vi "Oszilloscope_init.vi"(8 "error in":errorcluster, 11 "VISA-Ressourcenname":refnum<visa-resource-name>="USB0::0x0957::0x179B::MY54313507::INSTR") -> (0 "error out 2":errorcluster)   [LabVIEW 2016]
doc: "Mit diesem VI wird das Oszilloscope DSO-X-2002A initialisiert."
uses:
  <instrlib>/Agilent 2000 3000 X-Series/Agilent 2000 3000 X-Series.lvlib
panel:
  in  "Vertikale Skalierung (0,015 V/div)":dbl=0.015
  in  "Zeit Skalierung (0.004 Sec/div)":dbl=0.004
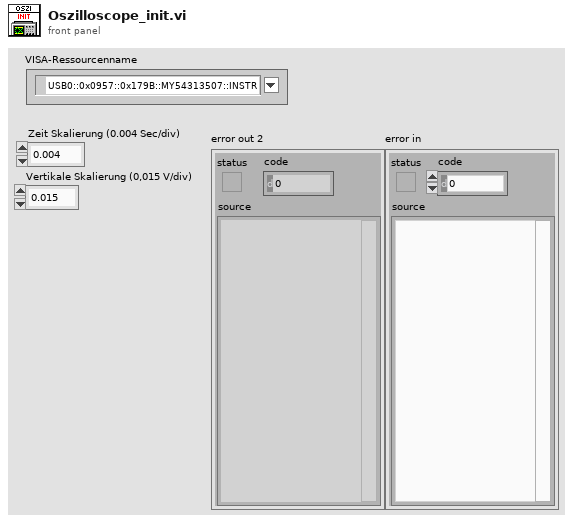
[diagram p1: front panel]
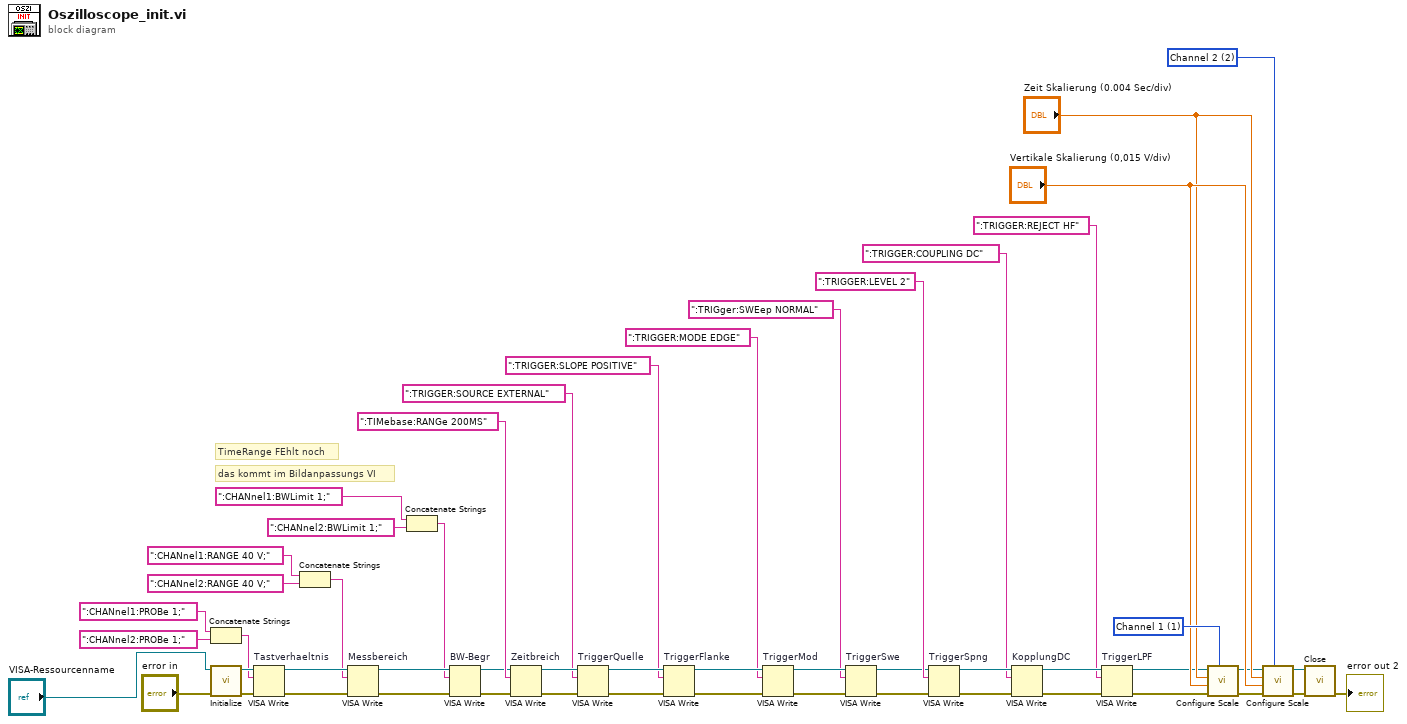
[diagram p0: block diagram]
diagram:
  w29 = 2 items=["Channel 1"=1, "Channel 2"=2, "Channel 3"=3, "Channel 4"=4] ("Channel Name (1: Channel 1)")
  w52 = 1 items=["Channel 1"=1, "Channel 2"=2, "Channel 3"=3, "Channel 4"=4] ("Channel Name (1: Channel 1)")
  # "das kommt im Bildanpassungs VI"
  # "TimeRange FEhlt noch"
  n1 = Concatenate Strings(":CHANnel1:PROBe 1;" ("Schreibpuffer"), ":CHANnel2:PROBe 1;" ("Schreibpuffer")) -> (w34:string)
  n2 = call <instrlib>:"Initialize.vi"("error in (no error)"="error in", "VISA resource name"="VISA-Ressourcenname") -> ("error out"=w48:errorcluster, "VISA resource name out"=w49:refnum<visa-resource-name>)  [unwired: 8 in]
  n3 = VISA Write "Tastverhaeltnis"(VISA resource name=w49, write buffer=w34, error in (no error)=w48) -> (VISA resource name out=w46:refnum<visa-resource-name>, error out=w43:errorcluster)  [unwired: 1 out]
  n4 = Concatenate Strings(":CHANnel1:RANGE 40 V;" ("Schreibpuffer"), ":CHANnel2:RANGE 40 V;" ("Schreibpuffer")) -> (w39:string)
  n5 = VISA Write "Messbereich"(VISA resource name=w46, write buffer=w39, error in (no error)=w43) -> (VISA resource name out=w45:refnum<visa-resource-name>, error out=w44:errorcluster)  [unwired: 1 out]
  n6 = Concatenate Strings(":CHANnel1:BWLimit 1;" ("Schreibpuffer"), ":CHANnel2:BWLimit 1;" ("Schreibpuffer")) -> (w40:string)
  n7 = VISA Write "BW-Begr"(VISA resource name=w45, write buffer=w40, error in (no error)=w44) -> (VISA resource name out=w28:refnum<visa-resource-name>, error out=w27:errorcluster)  [unwired: 1 out]
  n8 = VISA Write "Zeitbreich"(VISA resource name=w28, write buffer=":TIMebase:RANGe 200MS" ("Schreibpuffer"), error in (no error)=w27) -> (VISA resource name out=w20:refnum<visa-resource-name>, error out=w19:errorcluster)  [unwired: 1 out]
  n9 = VISA Write "TriggerQuelle"(VISA resource name=w20, write buffer=":TRIGGER:SOURCE EXTERNAL" ("Schreibpuffer"), error in (no error)=w19) -> (VISA resource name out=w24:refnum<visa-resource-name>, error out=w23:errorcluster)  [unwired: 1 out]
  n10 = VISA Write "TriggerFlanke"(VISA resource name=w24, write buffer=":TRIGGER:SLOPE POSITIVE" ("Schreibpuffer"), error in (no error)=w23) -> (VISA resource name out=w22:refnum<visa-resource-name>, error out=w21:errorcluster)  [unwired: 1 out]
  n11 = VISA Write "TriggerMod"(VISA resource name=w22, write buffer=":TRIGGER:MODE EDGE" ("Schreibpuffer"), error in (no error)=w21) -> (VISA resource name out=w8:refnum<visa-resource-name>, error out=w7:errorcluster)  [unwired: 1 out]
  n12 = VISA Write "TriggerSwe"(VISA resource name=w8, write buffer=":TRIGger:SWEep NORMAL" ("Schreibpuffer"), error in (no error)=w7) -> (VISA resource name out=w6:refnum<visa-resource-name>, error out=w5:errorcluster)  [unwired: 1 out]
  n13 = VISA Write "TriggerSpng"(VISA resource name=w6, write buffer=":TRIGGER:LEVEL 2" ("Schreibpuffer"), error in (no error)=w5) -> (VISA resource name out=w14:refnum<visa-resource-name>, error out=w13:errorcluster)  [unwired: 1 out]
  n14 = VISA Write "KopplungDC"(VISA resource name=w14, write buffer=":TRIGGER:COUPLING DC" ("Schreibpuffer"), error in (no error)=w13) -> (VISA resource name out=w17:refnum<visa-resource-name>, error out=w16:errorcluster)  [unwired: 1 out]
  n15 = VISA Write "TriggerLPF"(VISA resource name=w17, write buffer=":TRIGGER:REJECT HF" ("Schreibpuffer"), error in (no error)=w16) -> (VISA resource name out=w2:refnum<visa-resource-name>, error out=w3:errorcluster)  [unwired: 1 out]
  n16 = call <instrlib>:"Configure Scale.vi"("Channel Name (1: Channel 1)"=w52, "error in (no error)"=w3, "Vertical Scale (5 V/div)"="Vertikale Skalierung (0,015 V/div)", "Time Scale (0.0001 Sec/div)"="Zeit Skalierung (0.004 Sec/div)", "VISA resource name"=w2) -> ("error out"=w31:errorcluster, "VISA resource name out"=w30:refnum<visa-resource-name>)  [unwired: 5 in]
  n17 = call <instrlib>:"Configure Scale.vi"("Channel Name (1: Channel 1)"=w29, "error in (no error)"=w31, "Vertical Scale (5 V/div)"="Vertikale Skalierung (0,015 V/div)", "Time Scale (0.0001 Sec/div)"="Zeit Skalierung (0.004 Sec/div)", "VISA resource name"=w30) -> ("error out"=w25:errorcluster, "VISA resource name out"=w26:refnum<visa-resource-name>)  [unwired: 5 in]
  n18 = call <instrlib>:"Close.vi"("error in (no error)"=w25, "VISA resource name"=w26) -> ("error out"=→"error out 2":errorcluster)  [unwired: 9 in]
